vi "SetVirtualHostNameToFolderMapping.vi"(0 "reference in":refnum<class "DP_WebView.lvclass">=refnum, 1 "Host Folder":path=path "D:/GitProjects/LcANSUI/kendoui", 5 "error in (no error)":errorcluster, 6 "Access Type":i32(ring)=1 items=["Deny", "Allow", "DenyCors"]) -> (14 "reference out":refnum<class "DP_WebView.lvclass">, 19 "error out":errorcluster)   [LabVIEW 2020, in "DP_WebView.lvclass"]
uses:
  DP_WebView.lvclass
  C:/Projects/DependencyViewer/DependencyViewer/DP_WebView_class/data/Microsoft.Web.WebView2.Core.dll
  data/Microsoft.Web.WebView2.Core.dll
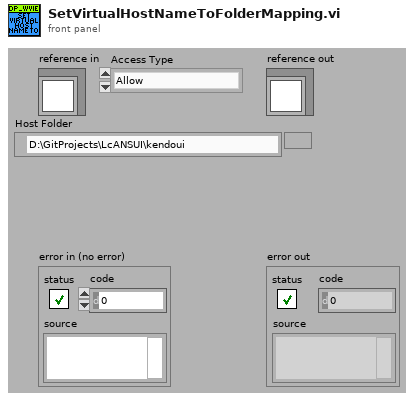
[diagram p1: front panel]
types:
  T1 = typedef "LcWebView.lvclass/ObjectAttributes.ctl" = cluster{"WebView Container":refnum<k24>, "CoreWebViewRef":refnum<k24>, "Status":i32, "Status Message":string, "User Data Folder":path, "BrowserProcessId":u32}
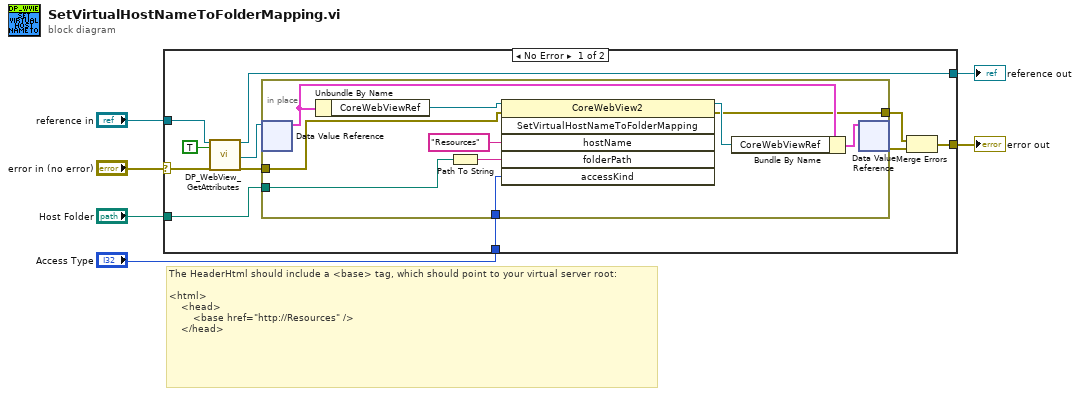
[diagram p0: block diagram]
diagram:
  # "The HeaderHtml should include a <base> tag, which should point to your virtual server root:\n\n<html>\n    <head>\n        <base href=\"http://Resources\" />\n    </head>"
  n1 = case shown="No Error" "error in (no error)" {
    selector: "error in (no error)" -> [w14 w29]
    tunnel: [w16 w29] -> w5
    tunnel: [w12 w28] -> w3
    tunnel: "reference in" -> [w15 w28]
    tunnel: "Host Folder" -> [w8 _]
    tunnel: "Access Type" -> [w7 _]
    frame No Error {
      n2 = call "DP_WebView_GetAttributes.vi"("reference in"=w15, "OnlyGetDvrReference(False)"=TRUE, "error in (no error)"=w14) -> ("reference out"=w12:refnum<class "DP_WebView.lvclass">, "DataRef"=w13:refnum<data-value>, "error out"=w10:errorcluster)  [unwired: 13 in, 1 out]
      n3 = in-place {
        in-place-border: w10 -> [w22]
        in-place-border: [w23] -> w9
        in-place-border: w8 -> [w20]
        in-place-border: w7 -> [w18]
        n4 = in-place-dvr #1(w13) -> (w26:T1)  [unwired: 1 out]
        n5 = Unbundle By Name(w26) -> ("CoreWebViewRef"=w25:refnum<k24>)
        n6 = Path To String(path=w20) -> (string=w19:string)
        n7 = invoke class="CoreWebView2" method="SetVirtualHostNameToFolderMapping"(reference=w25, error in=w22, "hostName"="Resources", "folderPath"=w19, "accessKind"=w18) -> (reference out=w24:refnum<k24>, error out=w23:errorcluster)  [unwired: 1 in, 4 out]
        n8 = Bundle By Name(cluster=w26, "CoreWebViewRef"=w24) -> (w27:T1)
        n9 = in-place-dvr #1(w27) -> (w17:errorcluster)  [unwired: 1 out]
      }
      n10 = Merge Errors(w9, w17) -> (w16:errorcluster)
    }
    frame Error {
    }
  }
  "error out" <- w5
  "reference out" <- w3
